vi "sub_format_datafile.vi"(10 "Dynamic data":T1) -> (2 "appended array":string[][](array[string]))   [LabVIEW 2020]
doc: "Arrange data in columns for output file."
uses:
  data_dynamic.ctl
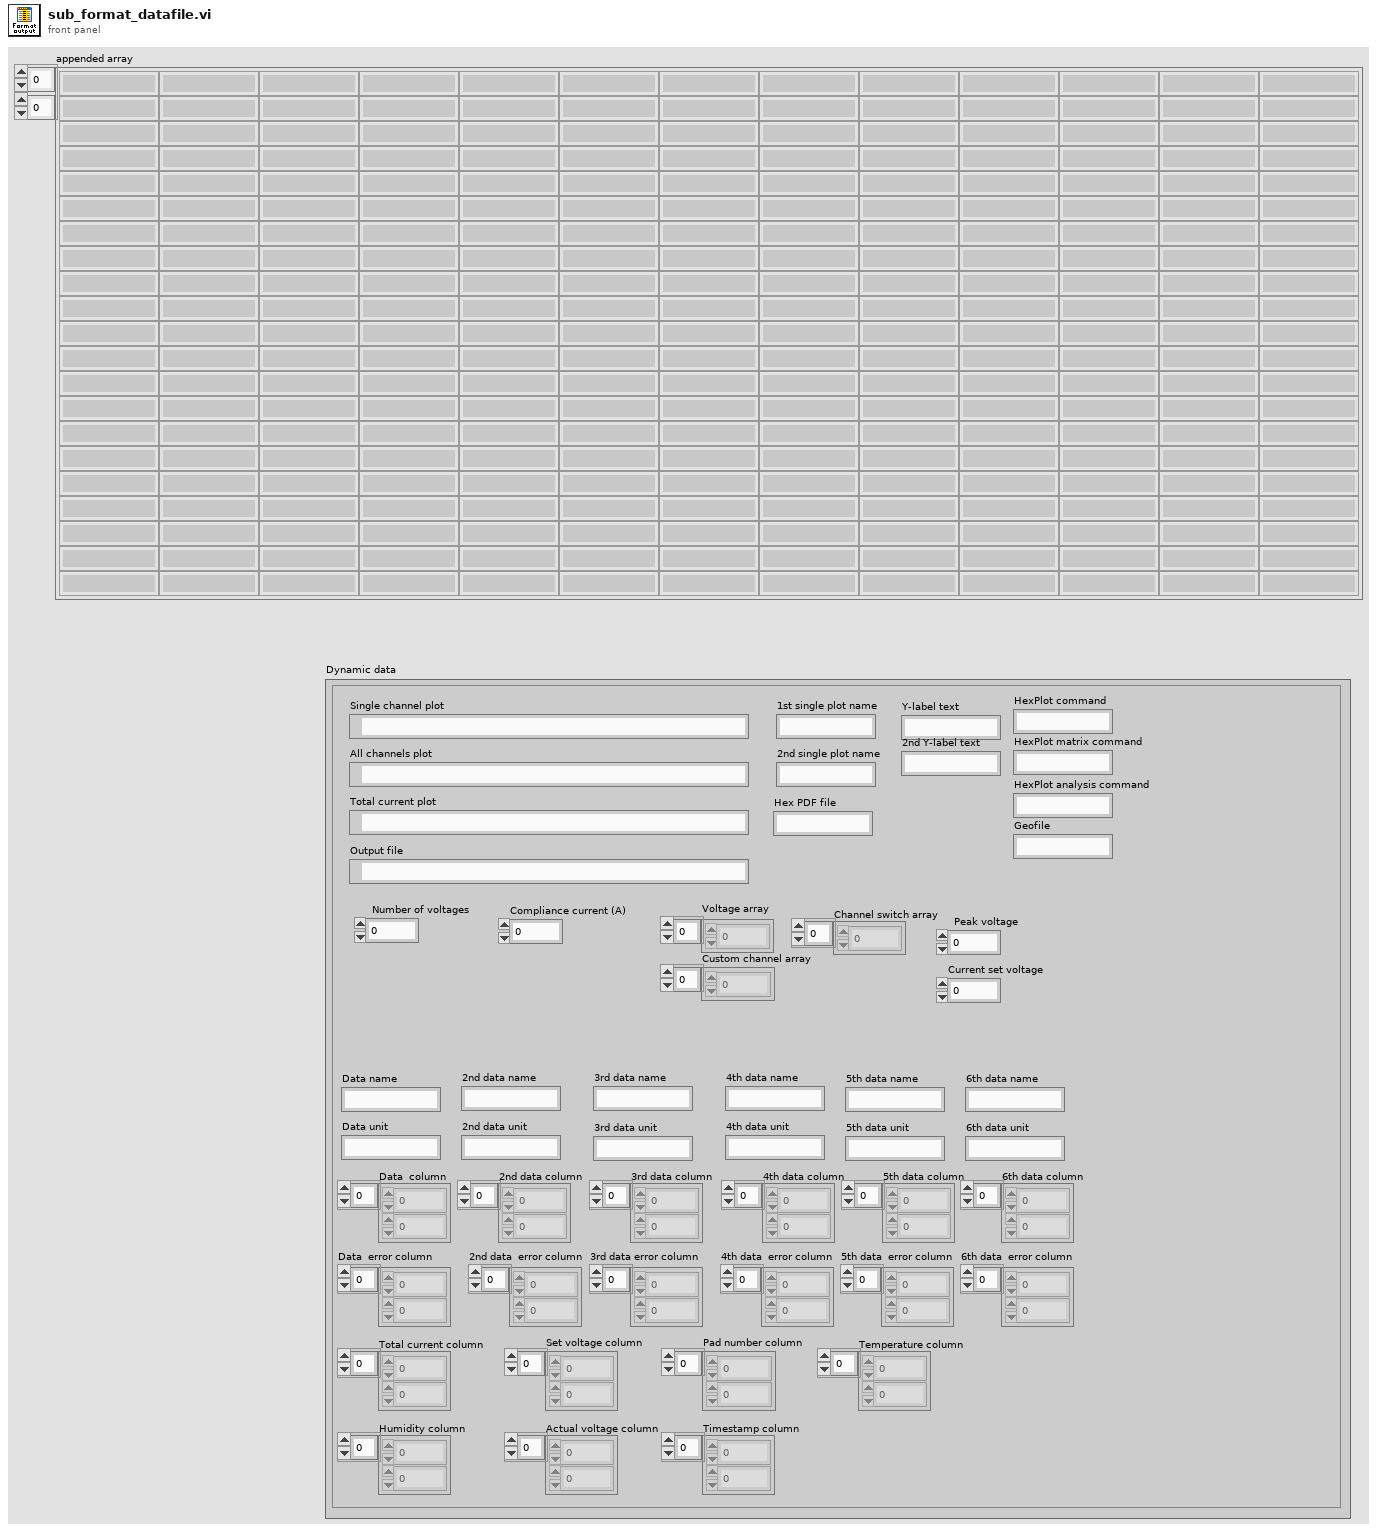
[diagram p1: front panel]
types:
  T1 = typedef "data_dynamic.ctl" = cluster{"Output file":path, "Y-label text":string, "Current set voltage":dbl, "Set voltage column":dbl[], "Pad number column":dbl[], "Data  column":dbl[], "Number of voltages":i32, "Compliance current (A)":dbl, "Geofile":string, "Peak voltage":dbl, "Hex PDF file":string, "Voltage array":dbl[], "Total current column":dbl[], "Timestamp column":dbl[], "Data name":string, "Data unit":string, "2nd data column":dbl[], "2nd data name":string, "2nd data unit":string, "3rd data column":dbl[], "4th data column":dbl[], "3rd data name":string, "3rd data unit":string, "4th data name":string, "4th data unit":string, "Actual voltage column":dbl[], "2nd Y-label text":string, "Single channel plot":path, "Temperature column":dbl[], "Humidity column":dbl[], "Channel switch array":i32[], "1st single plot name":string, "2nd single plot name":string, "All channels plot":path, "HexPlot command":string, "Custom channel array":i32[], "Data  error column":dbl[], "2nd data  error column":dbl[], "3rd data error column":dbl[], "4th data  error column":dbl[], "Total current plot":path, "5th data column":dbl[], "5th data  error column":dbl[], "6th data column":dbl[], "6th data  error column":dbl[], "5th data name":string, "5th data unit":string, "6th data name":string, "6th data unit":string, "HexPlot matrix command":string, "HexPlot analysis command":string}
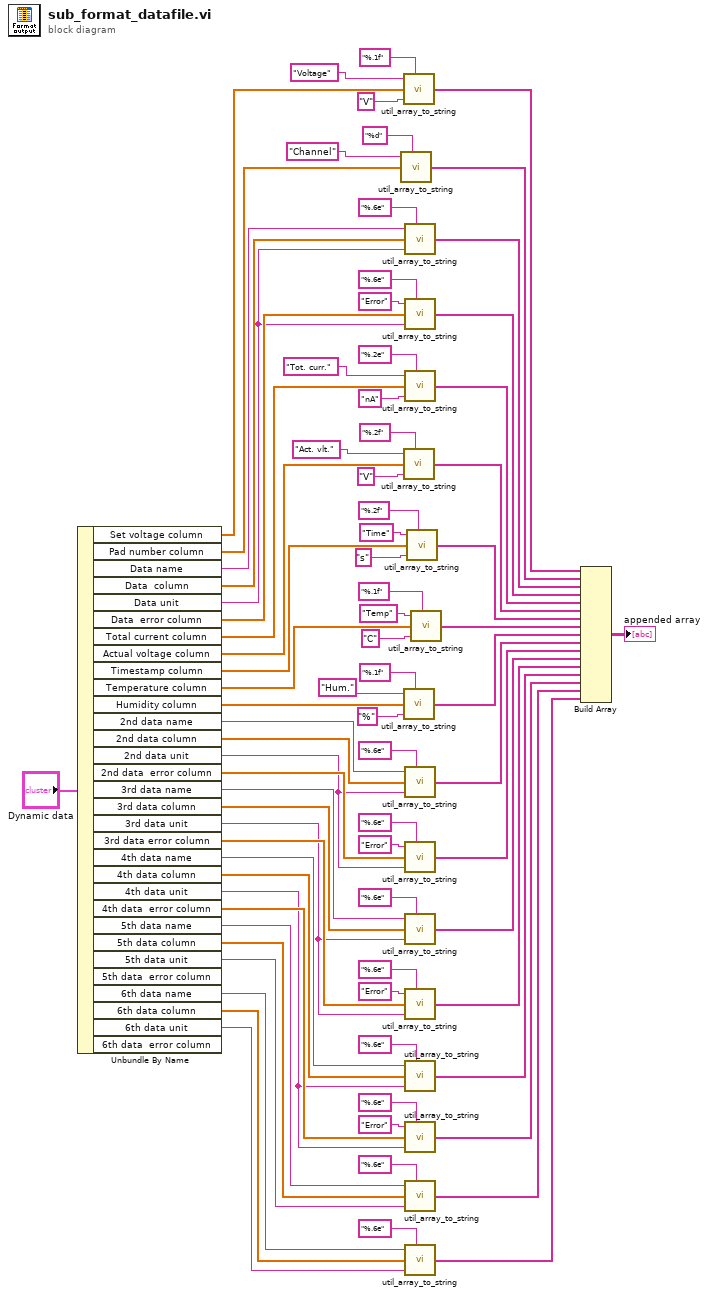
[diagram p0: block diagram]
diagram:
  n1 = Unbundle By Name("Dynamic data") -> ("Set voltage column"=w1:dbl[], "Pad number column"=w70:dbl[], "Data name"=w62:string, "Data  column"=w47:dbl[], "Data unit"=w29:string, "Data  error column"=w30:dbl[], "Total current column"=w69:dbl[], "Actual voltage column"=w43:dbl[], "Timestamp column"=w64:dbl[], "Temperature column"=w38:dbl[], "Humidity column"=w34:dbl[], "2nd data name"=w58:string, "2nd data column"=w54:dbl[], "2nd data unit"=w19:string, "2nd data  error column"=w20:dbl[], "3rd data name"=w53:string, "3rd data column"=w52:dbl[], "3rd data unit"=w17:string, "3rd data error column"=w18:dbl[], "4th data name"=w51:string, "4th data column"=w50:dbl[], "4th data unit"=w15:string, "4th data  error column"=w16:dbl[], "5th data name"=w9:string, "5th data column"=w7:dbl[], "5th data unit"=w8:string, "6th data name"=w6:string, "6th data column"=w5:dbl[], "6th data unit"=w4:string)  [unwired: 2 out]
  n2 = call "util_array_to_string.vi"("Header"="Channel", "Format"="%d", "Input 1D array"=w70) -> ("Output 1D array"=w76:string[])  [unwired: 6 in]
  n3 = call "util_array_to_string.vi"("Header"="Voltage", "Format"="%.1f", "Input 1D array"=w1, "Unit"="V") -> ("Output 1D array"=w77:string[])  [unwired: 5 in]
  n4 = call "util_array_to_string.vi"("Header"="Act. vlt.", "Format"="%.2f", "Input 1D array"=w43, "Unit"="V") -> ("Output 1D array"=w42:string[])  [unwired: 5 in]
  n5 = call "util_array_to_string.vi"("Header"="Hum.", "Format"="%.1f", "Input 1D array"=w34, "Unit"="%") -> ("Output 1D array"=w33:string[])  [unwired: 5 in]
  n6 = call "util_array_to_string.vi"("Header"=w62, "Format"="%.6e", "Input 1D array"=w47, "Unit"=w29) -> ("Output 1D array"=w78:string[])  [unwired: 5 in]
  n7 = call "util_array_to_string.vi"("Header"="Error", "Format"="%.6e", "Input 1D array"=w30, "Unit"=w29) -> ("Output 1D array"=w27:string[])  [unwired: 5 in]
  n8 = call "util_array_to_string.vi"("Header"="Tot. curr.", "Format"="%.2e", "Input 1D array"=w69, "Unit"="nA") -> ("Output 1D array"=w71:string[])  [unwired: 5 in]
  n9 = call "util_array_to_string.vi"("Header"=w58, "Format"="%.6e", "Input 1D array"=w54, "Unit"=w19) -> ("Output 1D array"=w57:string[])  [unwired: 5 in]
  n10 = call "util_array_to_string.vi"("Header"="Error", "Format"="%.6e", "Input 1D array"=w20, "Unit"=w19) -> ("Output 1D array"=w14:string[])  [unwired: 5 in]
  n11 = call "util_array_to_string.vi"("Header"=w53, "Format"="%.6e", "Input 1D array"=w52, "Unit"=w17) -> ("Output 1D array"=w49:string[])  [unwired: 5 in]
  n12 = call "util_array_to_string.vi"("Header"="Error", "Format"="%.6e", "Input 1D array"=w18, "Unit"=w17) -> ("Output 1D array"=w13:string[])  [unwired: 5 in]
  n13 = call "util_array_to_string.vi"("Header"=w51, "Format"="%.6e", "Input 1D array"=w50, "Unit"=w15) -> ("Output 1D array"=w48:string[])  [unwired: 5 in]
  n14 = call "util_array_to_string.vi"("Header"="Error", "Format"="%.6e", "Input 1D array"=w16, "Unit"=w15) -> ("Output 1D array"=w12:string[])  [unwired: 5 in]
  n15 = call "util_array_to_string.vi"("Header"=w9, "Format"="%.6e", "Input 1D array"=w7, "Unit"=w8) -> ("Output 1D array"=w3:string[])  [unwired: 5 in]
  n16 = call "util_array_to_string.vi"("Header"=w6, "Format"="%.6e", "Input 1D array"=w5, "Unit"=w4) -> ("Output 1D array"=w2:string[])  [unwired: 5 in]
  n17 = call "util_array_to_string.vi"("Header"="Time", "Format"="%.2f", "Input 1D array"=w64, "Unit"="s") -> ("Output 1D array"=w66:string[])  [unwired: 5 in]
  n18 = call "util_array_to_string.vi"("Header"="Temp", "Format"="%.1f", "Input 1D array"=w38, "Unit"="C") -> ("Output 1D array"=w32:string[])  [unwired: 5 in]
  n19 = Build Array(w77, w76, w78, w27, w71, w42, w66, w32, w33, w57, w14, w49, w13, w48, w12, w3, w2) -> (→"appended array":string[][])
